vi "rql_Set Sampling Config.vi"(4 "Show in Debugger?":bool=TRUE, 6 "Message Priority":T1=enum."Normal", 8 "error in":errorcluster, 10 "Data in":T2={"Sampling_Config"={"Fs"=1000.0, "#s"=1000.0}} {"Sampling_Config"."Fs" format="%.2p"}, 11 "Analog Signal in":refnum<class "Analog Signal.lvclass">) -> (0 "error out":errorcluster, 3 "dup Analog Signal out":refnum<class "Analog Signal.lvclass">)   [LabVIEW 2023, in "Analog Signal.lvclass"]
doc: "This VI sends a <b>Local API Request</b> message to an MHL case of the Worker that owns this VI.\n---\nSet sempling configuration of signal acquisition."
uses:
  Analog Signal.lvclass
  C:/Program Files (x86)/National Instruments/LabVIEW 2023/vi.lib/addons/_Workers/Library/Classes/Worker/Worker.lvclass
  rql_Set Sampling Config.ctl
  Support/Sampling Config.ctl
  <vilib>/addons/_Workers/Library/Classes/Message/Priority.ctl
  <vilib>/addons/_Workers/Library/Case Label.ctl
  <vilib>/addons/_Workers/Library/Classes/Message Queue/Message Queue.lvclass
  <vilib>/addons/_Workers/Library/Workers.lvlib
  <vilib>/addons/_Workers/Library/Classes/Message/Message.lvclass
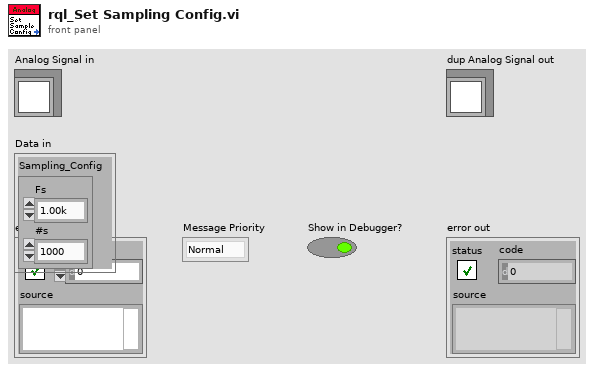
[diagram p1: front panel]
types:
  T1 = typedef "Workers.lvlib/Message.lvclass/Priority.ctl" = enum16{"Low", "Normal", "High"}
  T2 = typedef "Analog Signal.lvclass/rql_Set Sampling Config.ctl" = cluster{"Sampling_Config":T3}
  T3 = typedef "Analog Signal.lvclass/Sampling Config.ctl" = cluster{"Fs":dbl, "#s":dbl}
  T4 = typedef "Workers.lvlib/Case Label.ctl" = string
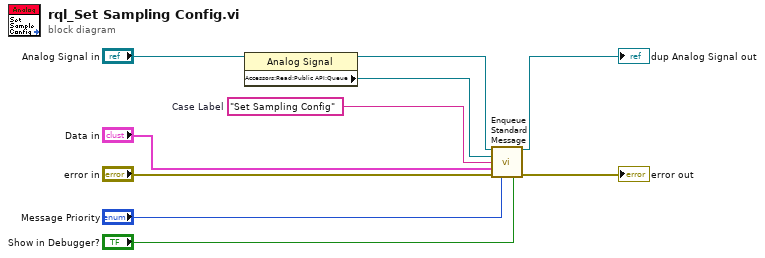
[diagram p0: block diagram]
diagram:
  w1 = T4 "Set Sampling Config"  # Case Label
  n1 = property class="Analog Signal"(reference="Analog Signal in") -> (reference out=w3:refnum<class "Analog Signal.lvclass">, "Accessors:Read:Public API:Queue"=w2:refnum<class "Message Queue.lvclass">)  [unwired: 1 in, 1 out]
  n2 = call-dynamic "Enqueue Standard Message.vi"("Worker"=w3, "Message Queue"=w2, "Case Label"=w1, "Data"="Data in", "error in (no error)"="error in", "Priority (Normal)"="Message Priority", "Send Message to Debugger? (T)"="Show in Debugger?") -> ("dup Worker out"=→"dup Analog Signal out":refnum<class "Analog Signal.lvclass">, "error out"=→"error out":errorcluster)  [unwired: 7 in]
